vi "Choreo_TrajectoryState_GetChassisSpeeds.vi"(11 "ChoreoTrajectoryState":T2) -> (3 "Chassis Speed":T1 {"vOmega" format="%10.3f"; "vY" format="%10.3f"; "vX" format="%10.3f"})   [LabVIEW 2019]
doc: "Return desired chassis speed from the trajectory state. This can be used as a feed forward for control.\n\nInputs:\n - ChoreoTrajectoryState - cluster - Individual trajectory state\n\nOutputs: \n - ChassisSpeeds - cluster - the field-relative chassis speeds of this state."
uses:
  TypeDef/ChoreoTrajectoryState.ctl
  <vilib>/Rock Robotics/WPI/ThirdParty/JAS_Junk/TrajLib/TypeDef/CHASSIS_SPEEDS.ctl
  <vilib>/Rock Robotics/WPI/ThirdParty/JAS_Junk/TrajLib/Trajectory_Library.lvlib
  ChoreoLib.lvlib
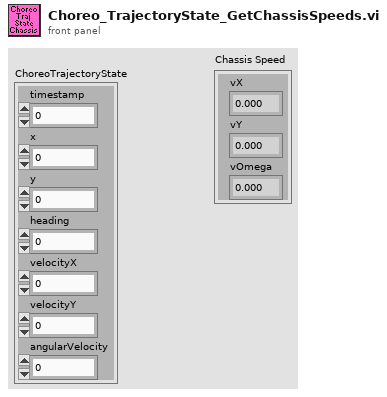
[diagram p1: front panel]
types:
  T1 = typedef "Trajectory_Library.lvlib/CHASSIS_SPEEDS.ctl" = cluster{"vX":dbl, "vY":dbl, "vOmega":dbl}
  T2 = typedef "ChoreoLib.lvlib/ChoreoTrajectoryState.ctl" = cluster{"timestamp":dbl, "x":dbl, "y":dbl, "heading":dbl, "velocityX":dbl, "velocityY":dbl, "angularVelocity":dbl}
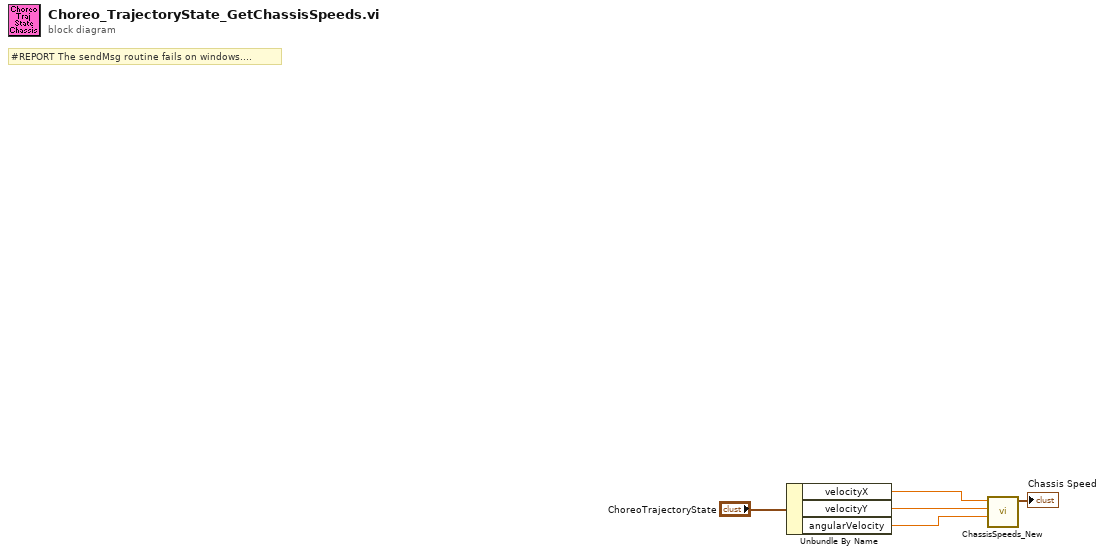
[diagram p0: block diagram]
diagram:
  # "#REPORT The sendMsg routine fails on windows...."
  n1 = Unbundle By Name("ChoreoTrajectoryState") -> ("velocityX"=w4:dbl, "velocityY"=w3:dbl, "angularVelocity"=w2:dbl)
  n2 = call <vilib>:"ChassisSpeeds_New.vi"("vAngular"=w2, "vY"=w3, "vX"=w4) -> ("CHASSIS"=→"Chassis Speed":T1)  [unwired: 8 in]
